vi "Update FPGA parameters.vi"(8 "error in (no error)":errorcluster, 11 "DAQ FPGA":T1={"Ref"=refnum, "Target"="RIO0", "Clock Freq (MHz) "=200.0, "input card type"=enum."AC Card", "Samples Wait after Trigger"=5080, "AOD fill"=4900, "StartupDelay"=0, "Slip Cycle (clock cycles)"=600000, "Add Cycle"=TRUE}) -> (0 "error out":errorcluster)   [LabVIEW 2013]
uses:
  Typedefs/DAQ FPGA config cluster.ctl
  RIG-SPECIFIC FILES/FPGA Refs/FPGA Ref.ctl
  <vilib>/userdefined/High Color/nirio_resource_hc.ctl
  Typedefs/FPGA input type AC-DC.ctl
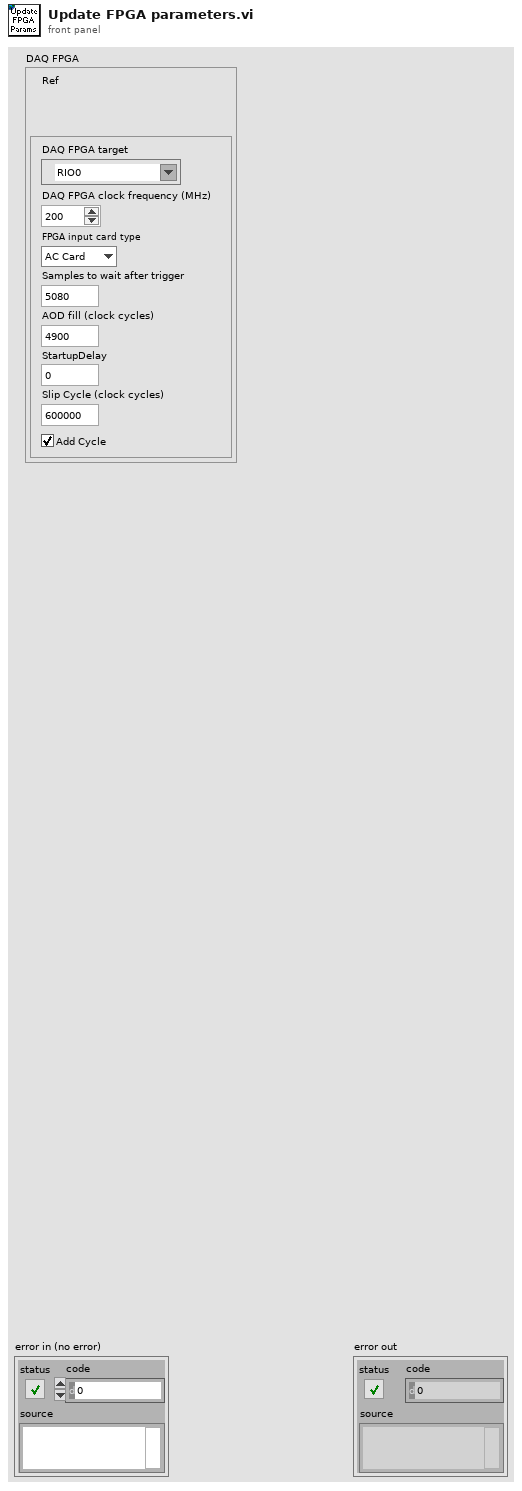
[diagram p1: front panel]
types:
  T1 = typedef "DAQ FPGA config cluster.ctl" = cluster{"Ref":T2, "Target":T3, "Clock Freq (MHz) ":dbl, "input card type":T4, "Samples Wait after Trigger":u16, "AOD fill":u16, "StartupDelay":i32, "Slip Cycle (clock cycles)":u32, "Add Cycle":bool}
  T2 = typedef "FPGA Ref.ctl" = refnum<k20>
  T3 = typedef "nirio_resource_hc.ctl" = tag
  T4 = typedef "FPGA input type AC-DC.ctl" = enum16{"AC Card", "DC Card"}
  T5 = typedef "AOL_Globals.ctl" = cluster{"Imaging Protocol":T6, "Number of POI":u16, "Number of Miniscans":u16, "Number of Trials":u16, "Number of Cycles ":u64, "# Averaged Frames":u16, "Laser power (%)":u8, "Pockels":dbl, "Acquisition Length (sec)":dbl, "Fill time (us)":dbl, "POI Dwell time (us)":dbl, "Miniscan Dwell time per pixel (us)":dbl, "PMT 1":dbl, "PMT 2":dbl, "Back Apperture":dbl, "Frame Size":T7, "Center Frequency":dbl, "Field of View":dbl, "DwellTime (us)":dbl, "Wavelength (nm)":dbl, "Zoom":dbl, "AOL Z":dbl, "AOL Mode":T8, "GridXY":dbl, "GridZ":dbl, "TriggerPeriod (sec)":dbl, "Number of Pixels in Miniscan":u16, "Experiment folder path":path, "X centre":dbl, "Y centre":dbl, "Angle (degrees)":dbl, "Plane Mode":T9, "Threshold":u16[], "Regenerate Chirps":bool, "Rectangle ROI length (pixels)":u16, "Rectangle ROI height (pixels)":u16, "AOD fill":u16, "Samples Wait after Trigger":u16, "StartUp Delay":i32, "Slip Cycle":u32, "Add Cycle":bool}
  T6 = typedef "Imaging Protocols enum.ctl" = enum16{"AOL Z-Stack", "Motor Z Stack", "Functional Acquisition", "Single Plane Acquisition", "Volume Acquisition", "Live Imaging", "Live Plane Imaging", "Live Volume Imaging"}
  T7 = typedef "Frame Size.ctl" = u16
  T8 = typedef "AOL modes.ctl" = enum16{"Raster", "Structural", "Pointing", "Mini Scan", "Alignment"}
  T9 = typedef "Plane Mode.ctl" = u16
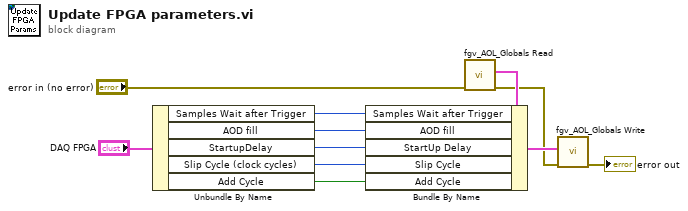
[diagram p0: block diagram]
diagram:
  n1 = Unbundle By Name("DAQ FPGA") -> ("Samples Wait after Trigger"=w7:u16, "AOD fill"=w8:u16, "StartupDelay"=w9:i32, "Slip Cycle (clock cycles)"=w10:u32, "Add Cycle"=w11:bool)
  n2 = call "fgv_AOL_Globals Read.vi"("error in (no error)"="error in (no error)") -> ("error out"=w3:errorcluster, "AOL_Globals"=w6:T5)  [unwired: 8 in, 1 out]
  n3 = Bundle By Name(cluster=w6, "Samples Wait after Trigger"=w7, "AOD fill"=w8, "StartUp Delay"=w9, "Slip Cycle"=w10, "Add Cycle"=w11) -> (w4:T5)
  n4 = call "fgv_AOL_Globals Write.vi"("error in (no error)"=w3, "AOL_Globals"=w4) -> ("error out"=→"error out":errorcluster)  [unwired: 9 in]
